vi "test_harness_hyst_sat_drift_parallel_fxp_16_5.vi"() -> ()   [LabVIEW 2019, in "Sat_Hyst_TestCase.lvclass"]
uses:
  Sat_Hyst_TestCase.lvclass
  C:/Program Files (x86)/National Instruments/LabVIEW 2019/vi.lib/addons/_JKI Toolkits/VI Tester/TestCase.llb/TestCase.lvclass
  <vilib>/rvi/DesktopExecutionNode/Execution/niFpgaDEN_Execute.vi
  <vilib>/rvi/DesktopExecutionNode/DesktopExecutionNode.xnode
  <vilib>/Wiresmith Technology/VITAC (VI Tester Advanced Comparisons)/VITAC.lvlib
panel:
  out "XY Graph":cluster{dbl[], dbl[]}[](graph)
  out "load-ticks":u32
  out "input cluster":T1
  in  "numIter":i32
  in  "error in (no error)":errorcluster
  out "error out":errorcluster
  out "TestCase out":refnum<class "Sat_Hyst_TestCase.lvclass">
  in  "TestCase in":refnum<class "Sat_Hyst_TestCase.lvclass">
  out "H_of_uk":fxp<+/-,32,10>[](array[numeric])
  out "sat(U) (expected, ML)":dbl[](array[numeric])
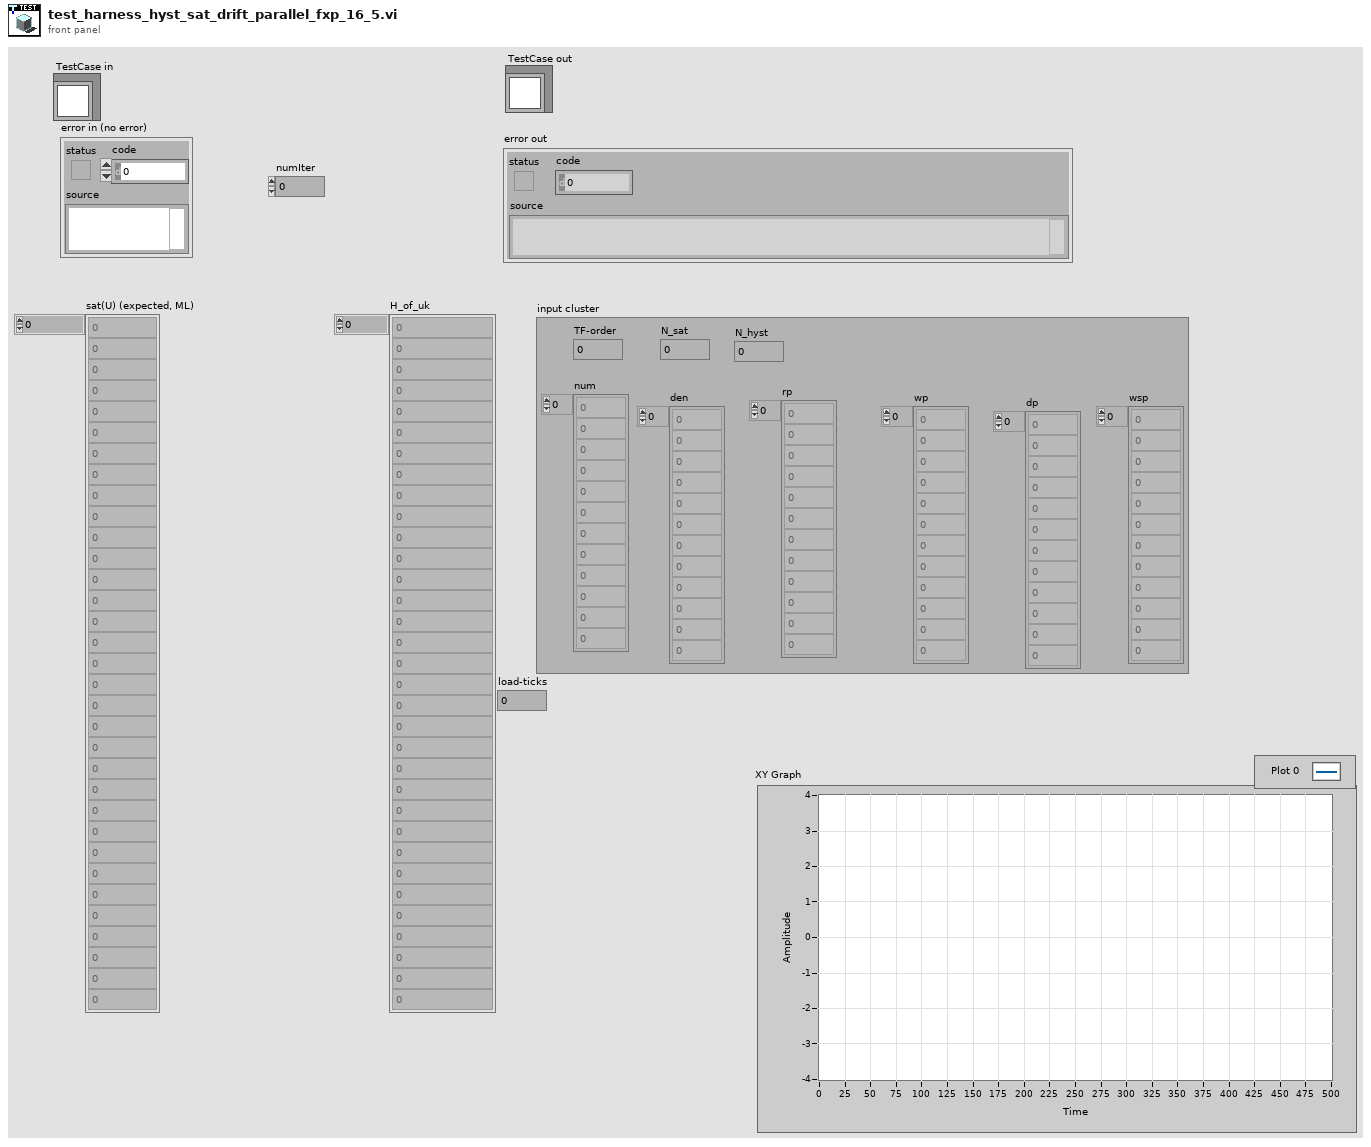
[diagram p1: front panel]
types:
  T1 = cluster{"TF-order":i32, "N_sat":i32, "N_hyst":i32, "num":dbl[], "wsp":dbl[], "dp":dbl[], "rp":dbl[], "wp":dbl[], "den":dbl[]}
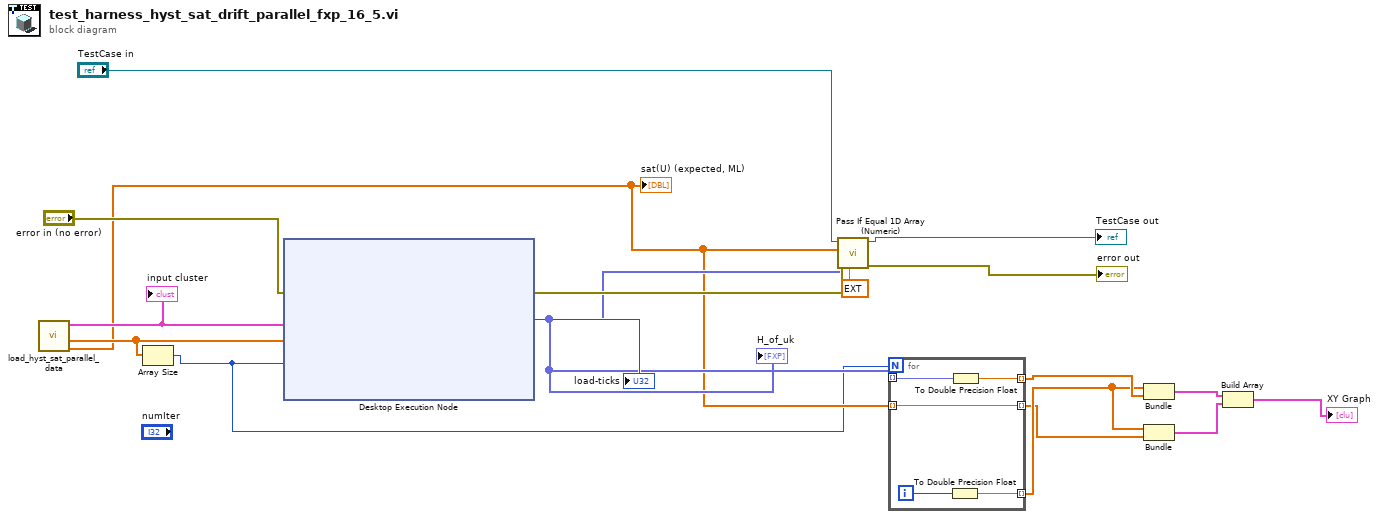
[diagram p0: block diagram]
diagram:
  n1 = call "load_hyst_sat_parallel_data.vi"() -> ("Hyst[U_nom]"=w8:dbl[], "U_nom"=w11:dbl[], "input cluster"=w12:T1)  [unwired: 9 in]
  "sat(U) (expected, ML)" <- w8
  "input cluster" <- w12
  n2 = Array Size(array=w11) -> (size(s)=w1:i32)
  n3 = xnode "Desktop Execution Node"("Error In"="error in (no error)", "input cluster"=w12, "uk"=w11, "numIter"=w1) -> ("Error Out"=w15:errorcluster, "H_of_uk"=w9:fxp<+/-,32,10>[], "load-ticks"=→"load-ticks":u32)
  "H_of_uk" <- w9
  n4 = call <vilib>:"Pass If Equal 1D Array (Numeric).vi"("delta (optional)"=ext 0.05, "error in (no error)"=w15, "actual"=w9, "expected"=w8, "TestCase in"="TestCase in") -> ("error out"=→"error out":errorcluster, "TestCase out"=→"TestCase out":refnum<class "Sat_Hyst_TestCase.lvclass">)  [unwired: 5 in]
  n5 = for {
    N: w1 -> [_]
    tunnel: w9 -> [w23] mode=indexing
    tunnel: [w22] -> w7 mode=indexing
    tunnel: [w21] -> w5 mode=indexing
    tunnel: w8 -> [w21] mode=indexing
    tunnel: [w20] -> w6 mode=indexing
    i -> [w19]
    n6 = To Double Precision Float(number=w19) -> (double precision float=w20:dbl)
    n7 = To Double Precision Float(number=w23) -> (double precision float=w22:dbl)
  }
  n8 = Bundle(w6, w7) -> (w4:cluster{dbl[], dbl[]})  [unwired: 1 in]
  n9 = Bundle(w6, w5) -> (w3:cluster{dbl[], dbl[]})  [unwired: 1 in]
  n10 = Build Array(w4, w3) -> (→"XY Graph":cluster{dbl[], dbl[]}[])
